vi "GV line clock change.vi"() -> ()   [LabVIEW 2017]
panel:
  in  "Line clock change":bool
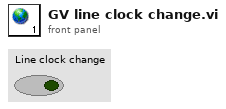
[diagram p1: front panel]
diagram:
